vi "get_y_middle_line.vi"(8 "error in (no error)":errorcluster, 11 "TrajectoryDL121017Hopping in":refnum<class "TrajectoryDL121017Hopping.lvclass">) -> (0 "error out":errorcluster, 2 "y middle line":dbl[unit], 3 "TrajectoryDL121017Hopping out":refnum<class "TrajectoryDL121017Hopping.lvclass">)   [LabVIEW 2010, in "TrajectoryDL121017Hopping.lvclass"]
doc: "Returns (in um) the mean of the maximum and the minimum y coordinate of all fix points."
uses:
  TrajectoryDL121017Hopping.lvclass
  TrajectoryDL121017Hopping.lvclass/TrajectoryDL121017Hopping.ctl
  common/classes/SpaceVector/SpaceVector/SpaceVector.lvclass
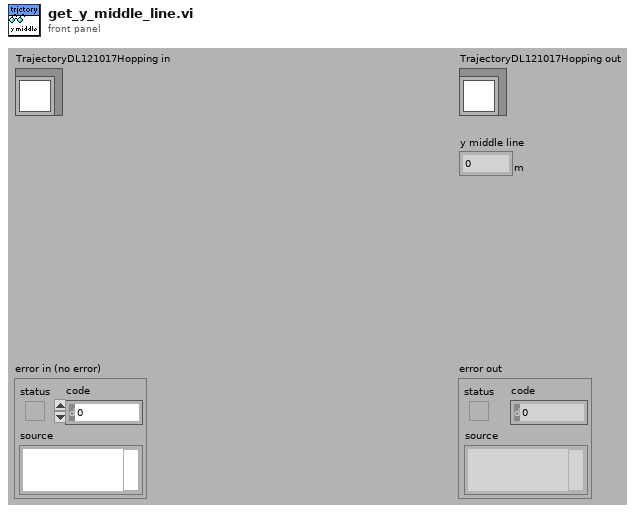
[diagram p1: front panel]
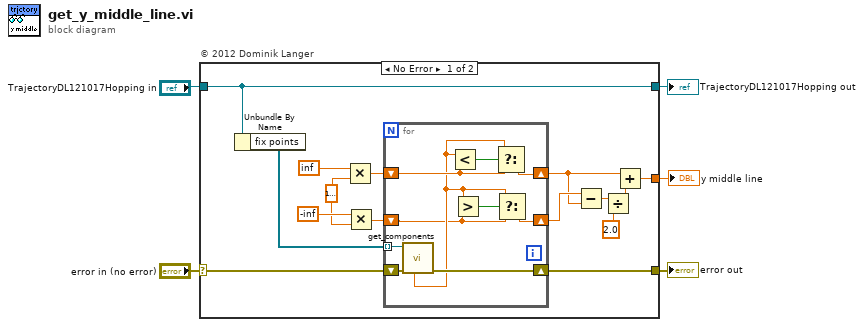
[diagram p0: block diagram]
diagram:
  n1 = case "© 2012 Dominik Langer" shown="No Error" "error in (no error)" {
    selector: "error in (no error)" -> [w9 w32]
    tunnel: [w8 w32] -> w2
    tunnel: [w7 w31] -> w5
    tunnel: "TrajectoryDL121017Hopping in" -> [w7 w31]
    tunnel: [w6 _] -> w1
    frame No Error {
      w17 = dbl[unit] 1e-06 ("y")
      n2 = Unbundle By Name(w7) -> ("fix points"=w20:refnum<class "SpaceVector.lvclass">[])
      n3 = Multiply(x=inf, y=w17) -> (x*y=w16:dbl[unit])
      n4 = Multiply(x=-inf, y=w17) -> (x*y=w15:dbl[unit])
      n5 = for {
        shift-right: [w28] -> w8
        shift-left: w9 -> [w30]
        tunnel: w20 -> [w29] mode=indexing
        shift-right: [w25] -> w11
        shift-left: w16 -> [w26]
        shift-right: [w23] -> w14
        shift-left: w15 -> [w21]
        n6 = call "get_components.vi"("error in (no error)"=w30, "SpaceVector in"=w29) -> ("error out"=w28:errorcluster, "y"=w22:dbl[unit])  [unwired: 4 in, 4 out]
        n7 = Less?(x=w22, y=w26) -> (x < y?=w27:bool)
        n8 = Greater?(x=w22, y=w21) -> (0:w24:bool)
        n9 = Select(t=w22, s=w27, f=w26) -> (s? t:f=w25:dbl[unit])
        n10 = Select(t=w22, s=w24, f=w21) -> (s? t:f=w23:dbl[unit])
      }
      n11 = Subtract(x=w14, y=w11) -> (x-y=w13:dbl[unit])
      n12 = Divide(x=w13, y=2.0) -> (x/y=w10:dbl[unit])
      n13 = Add(x=w11, y=w10) -> (x+y=w6:dbl[unit])
    }
    frame Error {
    }
  }
  "error out" <- w2
  "TrajectoryDL121017Hopping out" <- w5
  "y middle line" <- w1
